vi "Configure Modulation (Amplitude).vi"(0 "VISA resource name":refnum<visa-resource-name>, 1 "Modulation Frequency (1000 Hz)":dbl=1000.0, 2 "Modulation Depth (100 %)":i32=100, 5 "Enable Amplitude Modulation (T: Enable)":bool=TRUE, 7 "AM Source (0: Internal)":i32(ring) items=["Internal", "External"], 9 "Modulation Waveform (0: Sine)":i32(ring) items=["Sine", "Square", "Ramp", "Negative Ramp", "Triangle", "Noise", "Arbitrary Waveform"], 11 "error in (no error)":errorcluster) -> (4 "VISA resource name out":refnum<visa-resource-name>, 15 "error out":errorcluster)   [LabVIEW 2010, in "Agilent 33XXX Series.lvlib"]
doc: "Configures and enables amplitude modulation (AM). In AM, the amplitude of the carrier is varied by the amplitude of the modulating waveform. \n\nNote: The carrier waveform shape and parameters are set by the Configure Standard Waveform vi."
uses:
  <instrlib>/Agilent 33XXX Series/Agilent 33XXX Series.lvlib
panel:
  # "Internal AM Settings"
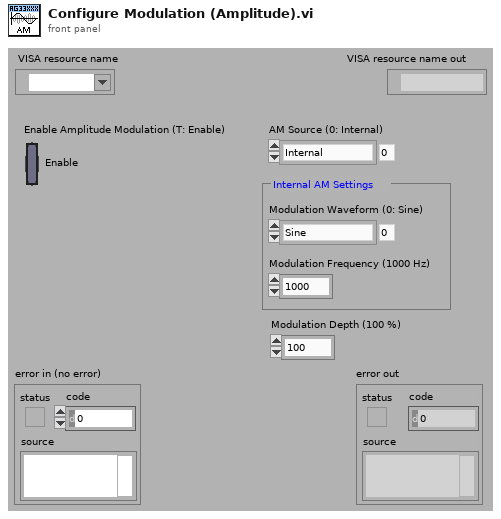
[diagram p1: front panel]
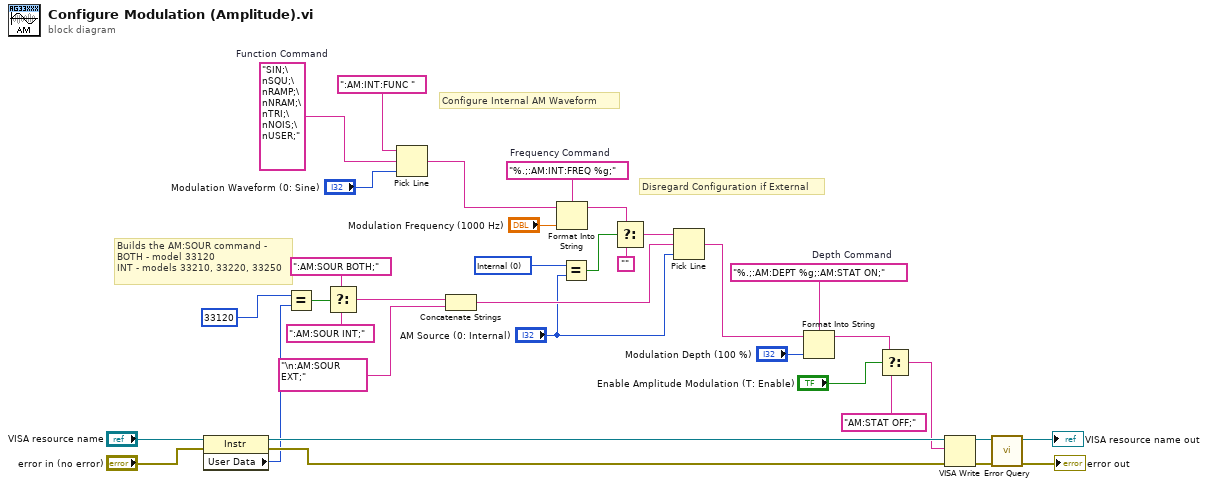
[diagram p0: block diagram]
diagram:
  w15 = "SIN;\nSQU;\nRAMP;\nNRAM;\nTRI;\nNOIS;\nUSER;"  # Function Command
  w17 = "%.;:AM:INT:FREQ %g;"  # Frequency Command
  w28 = "%.;:AM:DEPT %g;:AM:STAT ON;"  # Depth Command
  w7 = u16 0 items=["Internal", "External"] ("Source (0: Internal)")
  # "Disregard Configuration if External"
  # "Configure Internal AM Waveform"
  # "Builds the AM:SOUR command -\nBOTH - model 33120\nINT - models 33210, 33220, 33250"
  n1 = property class="Instr"(reference="VISA resource name", error in="error in (no error)") -> (reference out=w33:refnum<visa-resource-name>, error out=w32:errorcluster, "User Data"=w31:u32)
  n2 = Equal?(x=u32 33120, y=w31) -> (x = y?=w23:bool)
  n3 = Select(t=":AM:SOUR BOTH;", s=w23, f=":AM:SOUR INT;") -> (s? t:f=w20:string)
  n4 = Pick Line(string ("")=":AM:INT:FUNC ", multi-line string=w15, line index="Modulation Waveform (0: Sine)") -> (output string=w16:string)
  n5 = Concatenate Strings(w20, "\n:AM:SOUR EXT;" ("Source Command")) -> (w21:string)
  n6 = Format Into String(format string=w17, initial string=w16, "Modulation Frequency (1000 Hz)") -> (resulting string=w13:string)  [unwired: 1 in, 1 out]
  n7 = Equal?(x=w7, y="AM Source (0: Internal)") -> (x = y?=w8:bool)
  n8 = Select(t=w13, s=w8, f="") -> (s? t:f=w10:string)
  n9 = Pick Line(string ("")=w10, multi-line string=w21, line index="AM Source (0: Internal)") -> (output string=w9:string)
  n10 = Format Into String(format string=w28, initial string=w9, "Modulation Depth (100 %)") -> (resulting string=w18:string)  [unwired: 1 in, 1 out]
  n11 = Select(t=w18, s="Enable Amplitude Modulation (T: Enable)", f="AM:STAT OFF;") -> (s? t:f=w19:string)
  n12 = VISA Write(VISA resource name=w33, write buffer=w19, error in (no error)=w32) -> (VISA resource name out=w35:refnum<visa-resource-name>, error out=w34:errorcluster)  [unwired: 1 out]
  n13 = call <instrlib>:"Error Query.vi"("error in (no error)"=w34, "VISA resource name"=w35) -> ("error out"=→"error out":errorcluster, "VISA resource name out"=→"VISA resource name out":refnum<visa-resource-name>)  [unwired: 6 in, 2 out]
